vi "programa 12.vi"() -> ()   [LabVIEW 2011]
panel:
  in  "stop":bool
  in  "on/off":bool
  out "Foco":bool
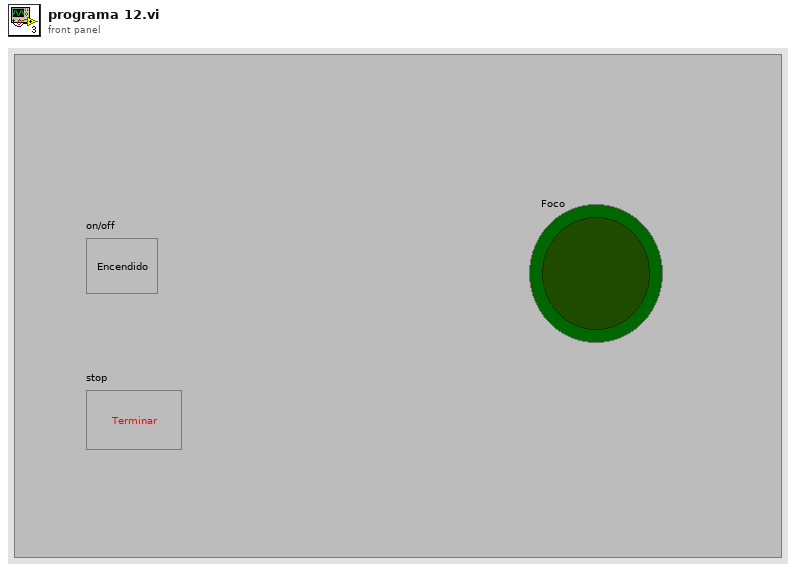
[diagram p1: front panel]
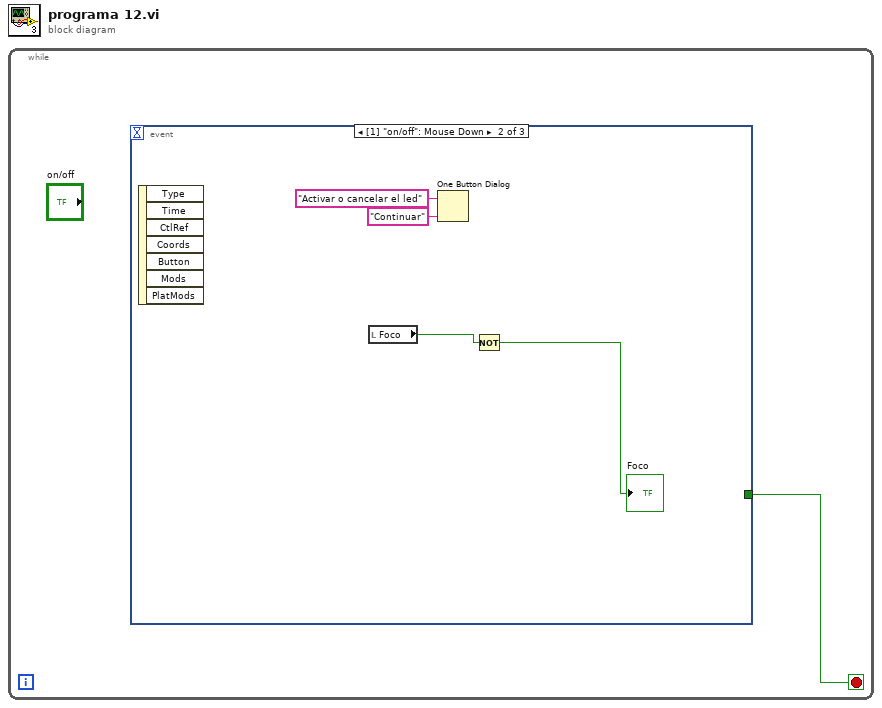
[diagram p0: block diagram]
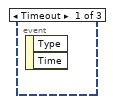
[diagram p2: hidden frame]
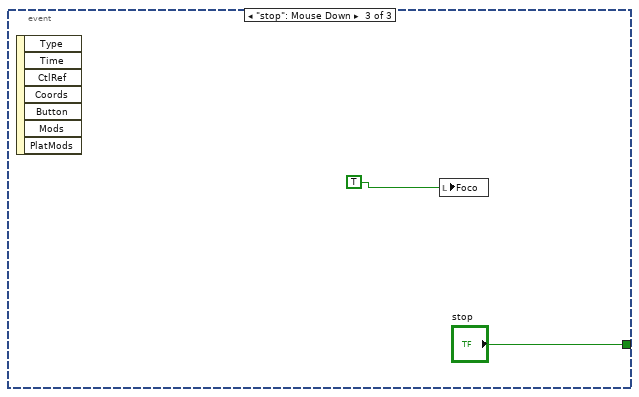
[diagram p3: hidden frame]
diagram:
  n1 = while {
    stop <- w1 stop-if-true
    n2 = event shown="[1] \"on/off\": Mouse Down" {
      selector: _ -> [_ _ _]
      dyn-events: _ -> [_ _ _]
      timeout: _ -> [_ _ _]
      tunnel: [_ _ "stop"] -> w1
      event Timeout {
        n3 = event-data() -> ()  [unwired: 1 in, 2 out]
      }
      event "on/off": Mouse Down {
        n4 = event-data() -> ()  [unwired: 1 in, 7 out]
        n5 = local read "Foco"() -> (w5:bool)
        n6 = One Button Dialog(message="Activar o cancelar el led", button name ("OK")="Continuar") -> ()  [unwired: 1 out]
        n7 = Not(x=w5) -> (.not. x?=→"Foco":bool)
      }
      event "stop": Mouse Down {
        n8 = event-data() -> ()  [unwired: 1 in, 7 out]
        n9 = local write "Foco"(TRUE) -> ()
      }
    }
  }
